vi "thermocouple.vi"() -> ()   [LabVIEW 2024]
panel:
  out "Scalar":dbl
  out "range":dbl
  out "Waveform Graph":dbl[](graph)
  in  "Stop":bool
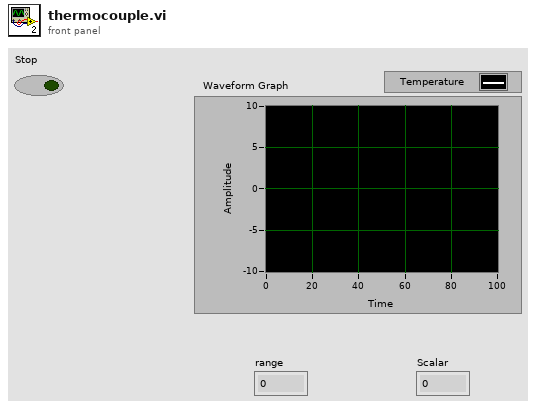
[diagram p1: front panel]
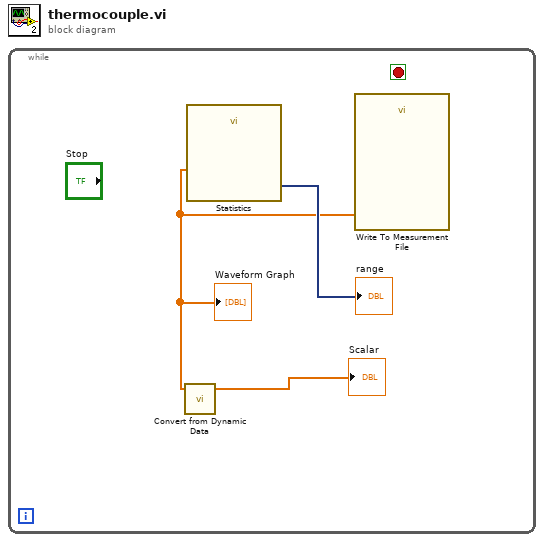
[diagram p0: block diagram]
diagram:
  n1 = while {
    stop <- _ stop-if-true
    n2 = call "Convert from Dynamic Data"("Dynamic Data Type"="Waveform Graph") -> ("Array"=→"Scalar":dbl[])  [unwired: 3 in]
    n3 = call "Statistics"("Signals"="Waveform Graph") -> ("Range"=→"range":dynamicdata)  [unwired: 25 in, 1 out]
    n4 = call "Write To Measurement File"("Signals"="Waveform Graph") -> ()  [unwired: 16 in, 3 out]
  }
